vi "Browser.vi"() -> ()   [LabVIEW 2023, in "LV-Awesome.lvlib"]
uses:
  LV-Awesome.lvlib
  LV Awesome/LV Awesome.lvclass/LV Awesome.ctl
  Freetype Drawer/Freetype Drawer/Freetype Drawer.lvclass
  LV Awesome/Read Fonts.vi
  LV Awesome/Read Glyphs.vi
  Font Glyph Drawer Interface/Bitmap Canvas/Bitmap Canvas.lvclass
  LV Awesome/LV Awesome.lvclass
  Font Glyph Drawer Interface/Transform/Transform.lvclass
  Glyph .NET Drawer/Drawer .Net.lvclass
  Font Glyph Drawer Interface/Glyph Canvas/Glyph Canvas.lvclass
panel:
  out "To":i32
  out "From":i32
  in  "Exit":bool
  in  "Namespace":string(combo)
  in  "Combo Box":string(combo) caption="Search"
  out "Count":i32 caption="# Results"
  in  "Scrollbar":i32(c297)
  out "Icons":T1(array[cluster])
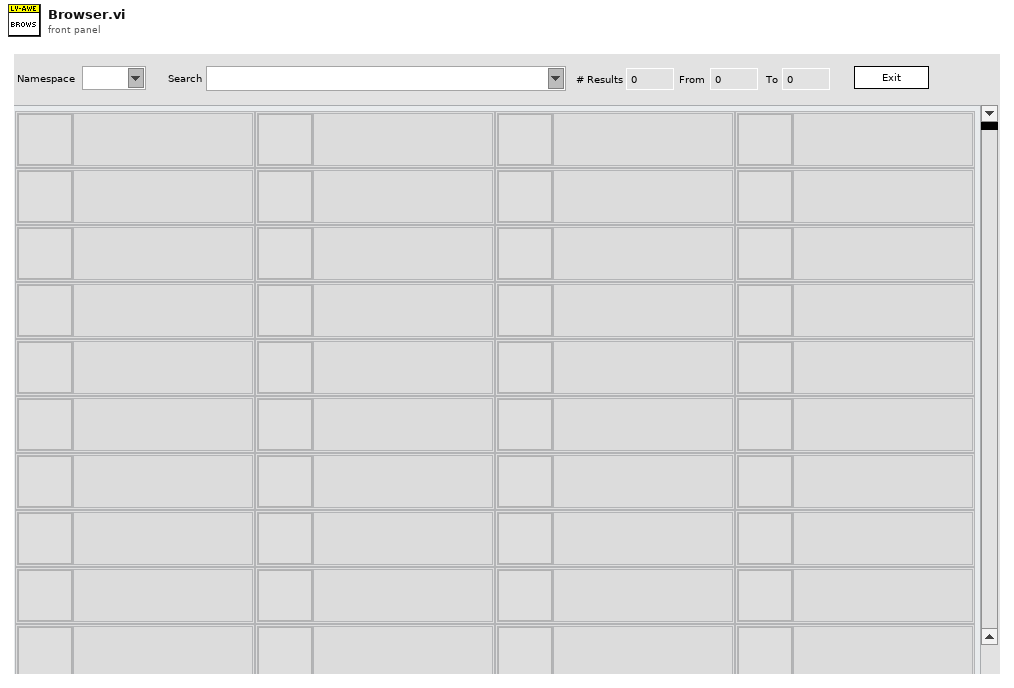
[diagram p1: front panel]
types:
  T1 = cluster{"2D Picture":picture, "String":string}[][]
  T2 = cluster{"Front":cluster{"Color":u32, "Alpha":u8}, "Back":cluster{"Color":u32, "Alpha":u8}}
  T3 = typedef "LVBoundsTypeDef.ctl" = cluster{"Width":u32, "Height":u32}
  T4 = cluster{"new picture":picture, "Glyph":string}[][]
  T5 = typedef "LVPoint32TypeDef.ctl" = cluster{"Horizontal":i32, "Vertical":i32}
  T6 = typedef "LVRowAndColumnTypeDef.ctl" = cluster{"Row":i32, "Column":i32}
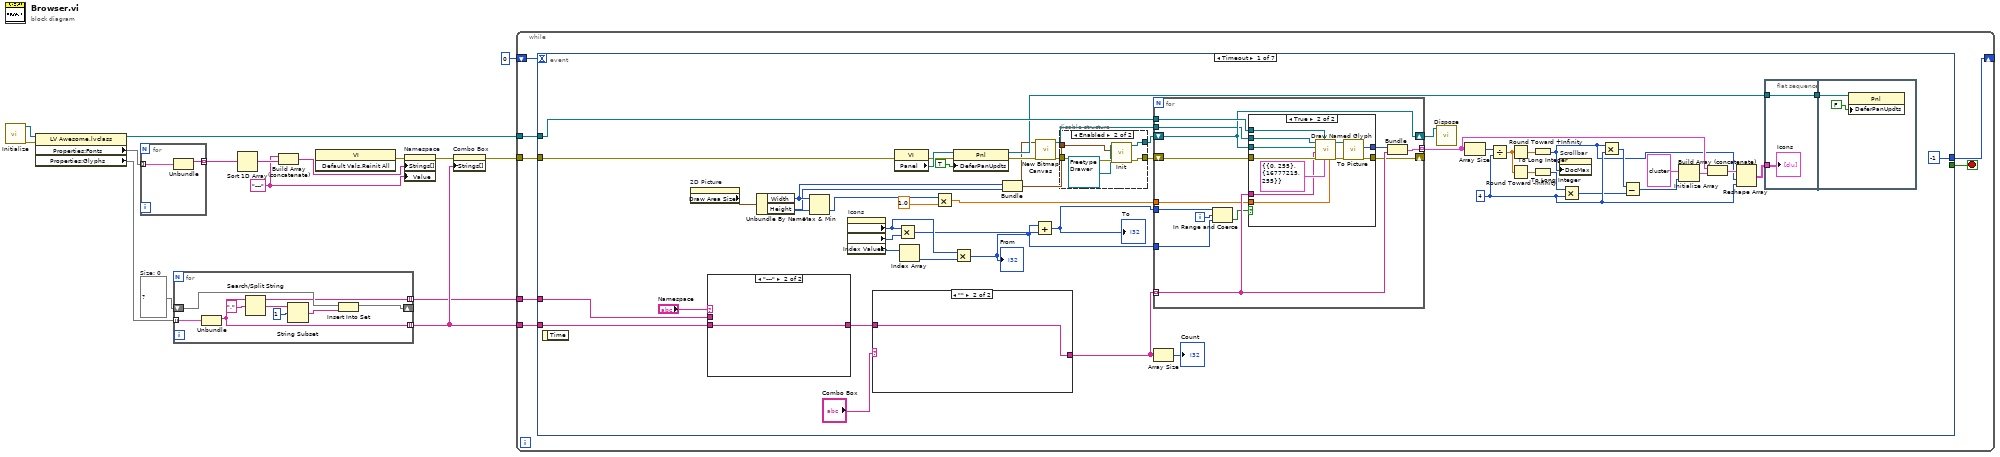
[diagram p0: block diagram]
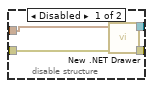
[diagram p2: hidden frame]
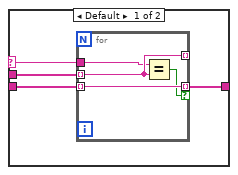
[diagram p3: hidden frame]
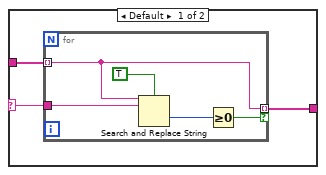
[diagram p4: hidden frame]
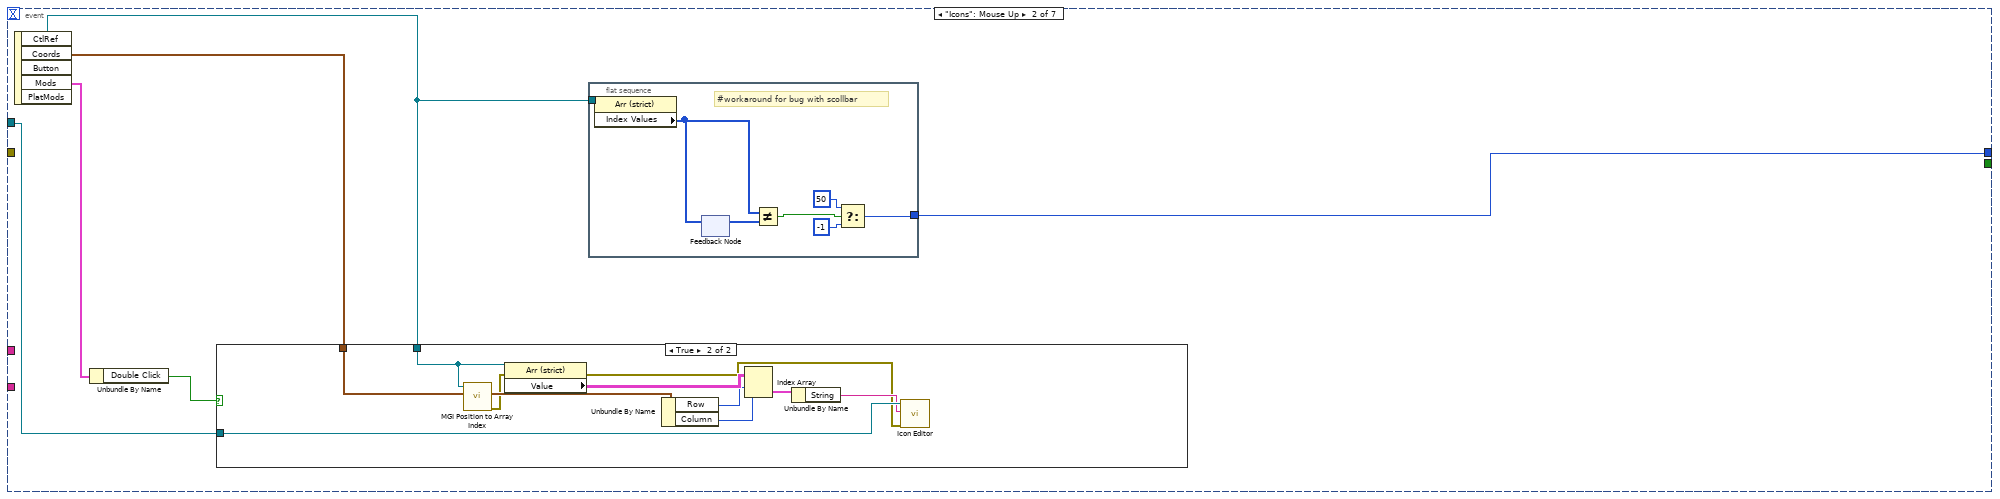
[diagram p6: hidden frame]
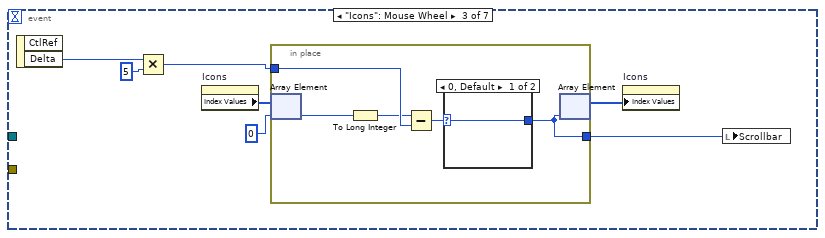
[diagram p8: hidden frame]
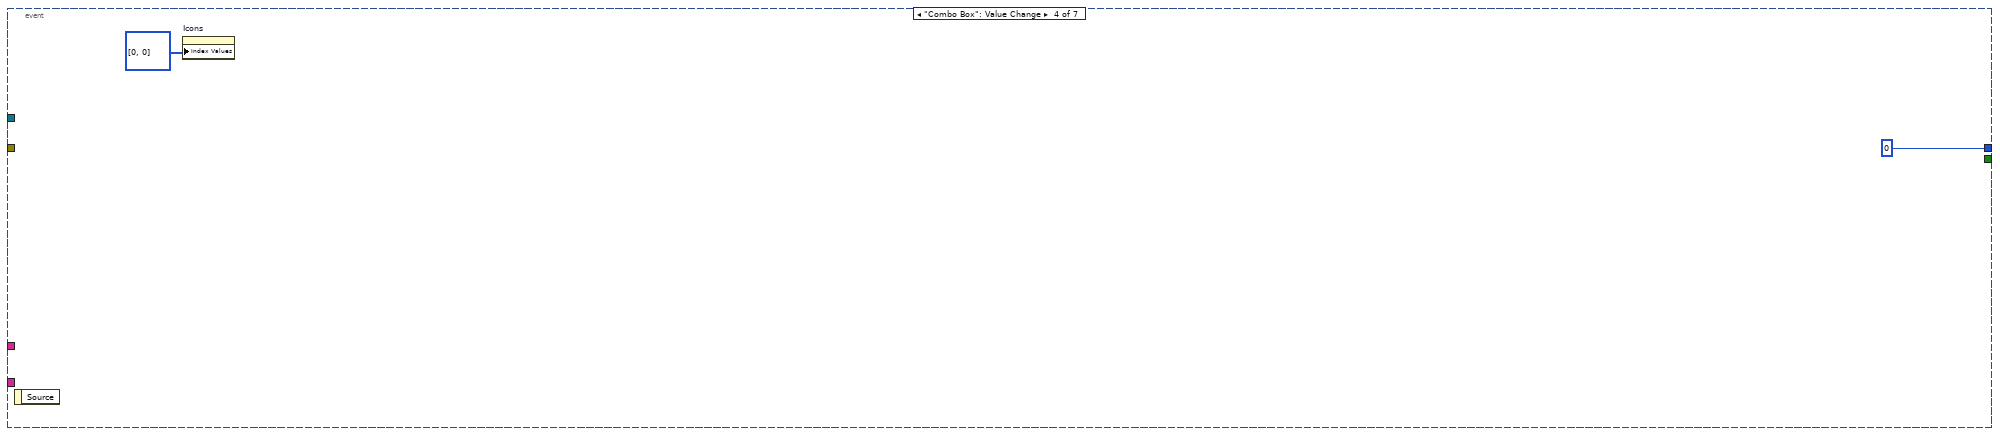
[diagram p10: hidden frame]
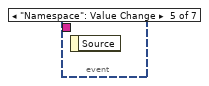
[diagram p11: hidden frame]
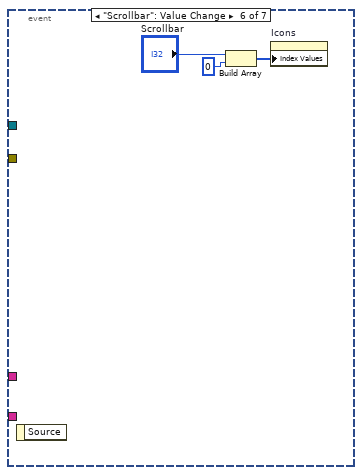
[diagram p12: hidden frame]
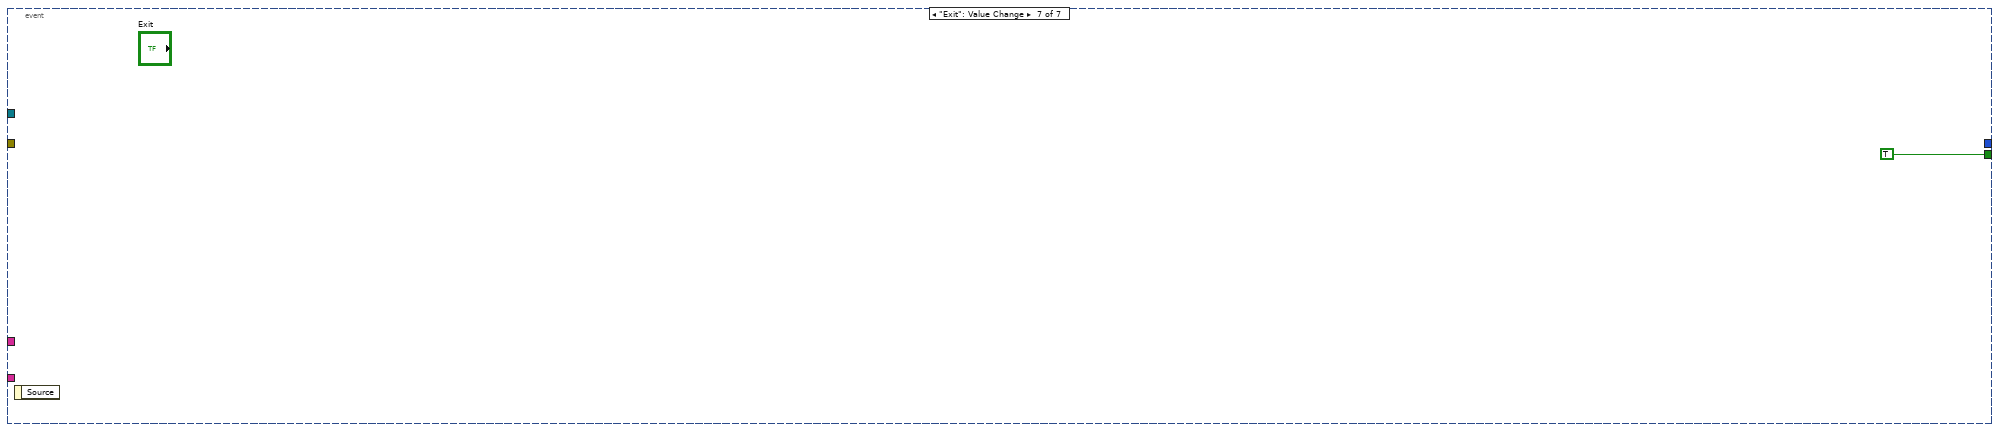
[diagram p13: hidden frame]
diagram:
  w8 = "---"
  w11 = set{string} {}  # Size: 0
  n1 = call "Initialize.vi"() -> ("error out"=w3:errorcluster, "LV Awesome"=w14:refnum<class "LV Awesome.lvclass">)  [unwired: 10 in]
  n2 = property class="LV Awesome.lvclass"(reference=w14, error in=w3) -> (reference out=w4:refnum<class "LV Awesome.lvclass">, "Properties:Fonts"=w2:map{string, path}, "Properties:Glyphs"=w1:map{string, u32})  [unwired: 1 out]
  n3 = for {
    tunnel: w2 -> [w18] mode=indexing
    tunnel: [w17] -> w13 mode=indexing
    n4 = Unbundle(w18) -> ("short"=w17:string)  [unwired: 1 out]
  }
  n5 = for {
    tunnel: w1 -> [w27] mode=indexing
    tunnel: [w26] -> w16 mode=indexing
    shift-right: [w21] -> _
    shift-left: w11 -> [w22]
    tunnel: [w19] -> w10 mode=indexing
    n6 = Unbundle(w27) -> ("Glyph"=w26:string)  [unwired: 1 out]
    n7 = Search/Split String(string=w26, search string/char (-)=".") -> (substring before match=w19:string, match + rest of string=w24:string)  [unwired: 1 in, 1 out]
    n8 = String Subset(string=w24, offset (0)=1) -> (substring=w20:string)  [unwired: 1 in]
    n9 = Insert Into Set(10:w20, 11:w22) -> (3:w21:set{string})  [unwired: 1 out]
  }
  n10 = Sort 1D Array(array=w13) -> (sorted array=w12:string[])
  n11 = Build Array (concatenate)(w8, w12) -> (w9:string[])
  n12 = invoke class="VI" method="Default Vals.Reinit All"() -> (error out=w7:errorcluster)  [unwired: 3 in, 2 out]
  n13 = property on="Namespace" class="CmbBox"(error in=w7, "Strings[]"=w9, "Value"=w8) -> (error out=w6:errorcluster)  [unwired: 1 in, 1 out]
  n14 = property on="Combo Box" class="CmbBox"(error in=w6, "Strings[]"=w16) -> (error out=w5:errorcluster)  [unwired: 1 in, 1 out]
  n15 = while {
    tunnel: w4 -> [w34]
    tunnel: w16 -> [w33]
    shift-right: [w31] -> _
    shift-left: 0 -> [w32]
    tunnel: w10 -> [w30]
    tunnel: w5 -> [w28]
    stop <- w29 stop-if-true
    n16 = event shown="[0] Timeout" {
      selector: _ -> [_ _ _ _ _ _ _]
      dyn-events: _ -> [_ _ _ _ _ _ _]
      timeout: w32 -> [_ _ _ _ _ _ _]
      tunnel: w34 -> [w84 w141 _ _ _ _ _]
      tunnel: w33 -> [w59 _ _ _ _ _ _]
      tunnel: [-1 w146 _ 0 _ _ _] -> w31
      tunnel: w30 -> [w57 _ _ _ _ _ _]
      tunnel: [_ _ _ _ _ _ TRUE] -> w29
      tunnel: w28 -> [w51 _ _ _ _ _ _]
      event Timeout {
        w66 = 4 ("y")
        n17 = event-data() -> ()  [unwired: 1 in, 1 out]
        n18 = property on="2D Picture" class="Pict"() -> ("Draw Area Size"=w40:T3)  [unwired: 2 in, 2 out]
        n19 = case shown="\"---\"" "Namespace" {
          selector: "Namespace" -> [w100 _]
          tunnel: w59 -> [w99 w106]
          tunnel: [w98 w106] -> w58
          tunnel: w57 -> [w101 _]
          frame Default {
            n20 = for {
              tunnel: [w105] -> _ mode=indexing
              tunnel: w101 -> [w105] mode=indexing
              tunnel: w100 -> [w104]
              tunnel: [w103] -> w98 mode=indexing if=w102
              tunnel: w99 -> [w103] mode=indexing
              n21 = Equal?(x=w104, y=w105) -> (x = y?=w102:bool)
            }
          }
          frame "---" {
          }
        }
        n22 = Unbundle By Name(w40) -> ("Width"=w36:u32, "Height"=w35:u32)
        n23 = Max & Min(x=w36, y=w35) -> (min(x,y)=w39:u32)  [unwired: 1 out]
        n24 = property on="Icons" class="Arr (strict)"() -> ("Number of Columns"=w78:u32, "Number of Rows"=w79:u32, "Index Values"=w81:u32[])  [unwired: 2 in, 2 out]
        n25 = case shown="\"\"" "Combo Box" {
          selector: "Combo Box" -> [w108 _]
          tunnel: w58 -> [w109 w115]
          tunnel: [w107 w115] -> w63
          frame Default {
            n26 = for {
              tunnel: w109 -> [w113] mode=indexing
              tunnel: w108 -> [w114]
              tunnel: [w113] -> w107 mode=indexing if=w111
              n27 = Search and Replace String(case sensitive?=TRUE ("ignore case? (F)"), input string=w113, search string=w114) -> (offset past replacement=w112:i32)  [unwired: 5 in, 3 out]
              n28 = Greater Or Equal To 0?(x=w112) -> (x >= 0?=w111:bool)
            }
          }
          frame "" {
          }
        }
        n29 = property class="VI"(error in=w51) -> (error out=w48:errorcluster, "Panel"=w50:refnum<vi>)  [unwired: 1 in, 1 out]
        n30 = Multiply(x=w78, y=w79) -> (x*y=w77:u32)
        n31 = Index Array(array=w81) -> (element=w80:u32)  [unwired: 1 in]
        n32 = Multiply(x=w39, y=1.0) -> (x*y=w38:dbl)
        n33 = property class="Pnl"(reference=w50, error in=w48, "DeferPanUpdts"=TRUE ("Defer Panel Updates")) -> (reference out=w44:refnum<vi>, error out=w47:errorcluster)
        n34 = Multiply(x=w78, y=w80) -> (x*y=w54:u32)
        "From" <- w54
        n35 = Bundle("Width"=w36, "Height"=w35) -> (w41:cluster{"Width":u32, "Height":u32})  [unwired: 1 in]
        n36 = Add(x=w54, y=w77) -> (x+y=w53:u32)
        "To" <- w53
        n37 = call "New Bitmap Canvas.vi"("error in (no error)"=w47, "Size"=w41) -> ("error out"=w46:errorcluster, "Bitmap Canvas out"=w52:refnum<class "Bitmap Canvas.lvclass">)  [unwired: 8 in]
        n38 = disable-structure shown="Enabled" {
          disable-tunnel: [w88 w90] -> w62
          disable-tunnel: w46 -> [w87 w93]
          disable-tunnel: [w86 w92] -> w45
          disable-tunnel: w41 -> [w85 w89]
          frame Disabled {
            n39 = call "New .NET Drawer.vi"("error in (no error)"=w87, "Size"=w85) -> ("error out"=w86:errorcluster, "Canvas out"=w88:refnum<class "Drawer .Net.lvclass">)  [unwired: 8 in]
          }
          frame Enabled {
            n40 = call-dynamic "Init.vi"("error in (no error)"=w93, "Size"=w89, "Class 1 in"=refnum<class "Freetype Drawer.lvclass"> refnum ("Freetype Drawer.lvlib:Freetype Drawer.lvclass")) -> ("error out"=w92:errorcluster, "Class 1 out"=w90:refnum<class "Freetype Drawer.lvclass">)  [unwired: 7 in]
          }
        }
        n41 = for {
          tunnel: [w127] -> w76 mode=indexing
          tunnel: w84 -> [w126]
          tunnel: w63 -> [w125] mode=indexing
          tunnel: w54 -> [w122]
          tunnel: w53 -> [w121]
          tunnel: w38 -> [w119]
          tunnel: w52 -> [w118]
          shift-right: [w117] -> _
          shift-left: w45 -> [w116]
          shift-right: [w124] -> w61
          shift-left: w62 -> [w124]
          i -> [w123]
          n42 = In Range and Coerce(upper limit=w121, x=w123, lower limit=w122) -> (In Range?=w120:bool)  [unwired: 1 out]
          n43 = case shown="True" w120 {
            tunnel: [_ w140] -> w128
            tunnel: w126 -> [_ w133]
            tunnel: w125 -> [_ w132]
            tunnel: w124 -> [_ w139]
            tunnel: w119 -> [_ w130]
            tunnel: w118 -> [_ w138]
            tunnel: [w129 w137] -> w117
            tunnel: w116 -> [w129 w134]
            frame False {
            }
            frame True {
              n44 = call "Draw Named Glyph.vi"("Size"=w130, "Colors"=T2 {"Front"={"Color"=0, "Alpha"=255}, "Back"={"Color"=16777215, "Alpha"=255}}, "Glyph Source in"=w133, "error in (no error)"=w134, "Glyph Name"=w132, "Glyph Drawer in"=w139, "Glyph Canvas in"=w138) -> ("error out"=w136:errorcluster, "Glyph Canvas out"=w131:refnum<class "Bitmap Canvas.lvclass">)  [unwired: 2 in, 1 out]
              n45 = call "To Picture.vi"("error in (no error)"=w136, "Bitmap Canvas in"=w131) -> ("error out"=w137:errorcluster, "new picture"=w140:picture)  [unwired: 7 in, 1 out]
            }
          }
          n46 = Bundle("new picture"=w128, "Glyph"=w125) -> (w127:cluster{"new picture":picture, "Glyph":string})  [unwired: 1 in]
        }
        n47 = Array Size(array=w63) -> (size(s)=→"Count":i32)
        n48 = call-dynamic "Dispose.vi"("Class 1 in"=w61) -> ()  [unwired: 10 in, 1 out]
        n49 = Array Size(array=w76) -> (size(s)=w75:i32)
        n50 = Divide(x=w75, y=w66) -> (x/y=w69:dbl)
        n51 = Round Toward +Infinity(x=w69) -> (ceil(x): smallest int >= x=w70:dbl)
        n52 = Round Toward -Infinity(1:w69) -> (0:w68:dbl)
        n53 = To Long Integer(number=w70) -> (32bit integer=w55:i32)
        n54 = To Long Integer(number=w68) -> (32bit integer=w67:i32)
        n55 = property on="Scrollbar" class="Scroll (strict)"("DocMax"=w55) -> ()  [unwired: 2 in, 2 out]
        n56 = Multiply(x=w67, y=w66) -> (x*y=w64:i32)
        n57 = Multiply(x=w55, y=w66) -> (x*y=w65:i32)
        n58 = Subtract(x=w65, y=w64) -> (x-y=w71:i32)
        n59 = Initialize Array(cluster{"new picture":picture, "Glyph":string} {"new picture"=bytes[0], "Glyph"=""}, w71) -> (w72:cluster{"new picture":picture, "Glyph":string}[])
        n60 = Build Array (concatenate)(w76, w72) -> (w73:cluster{"new picture":picture, "Glyph":string}[])
        n61 = Reshape Array(w73, w55, w66) -> (w42:T4)
        n62 = flat-sequence {
          tunnel: w44 -> [w95]
          tunnel: [w95] -> w43
          tunnel: w42 -> [w94]
          tunnel: w43 -> [w97]
          frame #0 {
            "Icons" <- w94
          }
          frame #1 {
            n63 = property class="Pnl"(reference=w97, "DeferPanUpdts"=FALSE ("Defer Panel Updates")) -> ()  [unwired: 1 in, 2 out]
          }
        }
      }
      event "Icons": Mouse Up {
        n64 = event-data() -> ("CtlRef"=w144:refnum<vi>, "Coords"=w142:T5, "Mods"=w145:cluster{"Double Click":bool, "Menu Key":bool})  [unwired: 1 in, 2 out]
        n65 = Unbundle By Name(w145) -> ("Double Click"=w143:bool)
        n66 = case shown="True" w143 {
          tunnel: w144 -> [_ w155]
          tunnel: w142 -> [_ w157]
          tunnel: w141 -> [_ w150]
          frame False {
          }
          frame True {
            n67 = call <userlib>:"MGI Position to Array Index.vi"("Coords"=w157, "ArrayRef"=w155) -> ("error out"=w147:errorcluster, "Index"=w156:T6)  [unwired: 5 in, 3 out]
            n68 = property class="Arr (strict)"(reference=w155, error in=w147) -> (error out=w148:errorcluster, "Value"=w154:T1)  [unwired: 1 out]
            n69 = Unbundle By Name(w156) -> ("Row"=w153:i32, "Column"=w152:i32)
            n70 = Index Array(array=w154, index (row)=w153, index (col)=w152) -> (element=w151:cluster{"2D Picture":picture, "String":string})
            n71 = Unbundle By Name(w151) -> ("String"=w149:string)
            n72 = call "Icon Editor.vi"("error in (no error)"=w148, "Glyph"=w149, "Glyph Source in"=w150) -> ()  [unwired: 7 in, 2 out]
          }
        }
        n73 = flat-sequence {
          tunnel: w144 -> [w164]
          tunnel: [w163] -> w146
          frame #0 {
            # "#workaround for bug with scollbar"
            n74 = property class="Arr (strict)"(reference=w164) -> ("Index Values"=w161:u32[])  [unwired: 1 in, 2 out]
            n75 = feedback #1() -> (w162:u32[])  [unwired: 1 in]
            n76 = feedback-in #1(w161) -> ()
            n77 = Not Equal?(x=w161, y=w162) -> (x != y?=w159:bool)
            n78 = Select(t=50, s=w159, f=-1) -> (s? t:f=w163:i32)
          }
        }
      }
      event "Icons": Mouse Wheel {
        n79 = event-data() -> ("Delta"=w171:i32)  [unwired: 1 in, 1 out]
        n80 = Multiply(x=w171, y=5) -> (x*y=w167:i32)
        n81 = property on="Icons" class="Arr (strict)"() -> ("Index Values"=w170:u32[])  [unwired: 2 in, 2 out]
        n82 = in-place {
          in-place-border: w167 -> [w175]
          in-place-border: [w172] -> w165
          n83 = in-place-array #2(w170, 0) -> (w176:u32)
          n84 = To Long Integer(number=w176) -> (32bit integer=w174:i32)
          n85 = Subtract(x=w174, y=w175) -> (x-y=w173:i32)
          n86 = case shown="0, Default" w173 {
            selector: w173 -> [w177 _]
            tunnel: [w177 _] -> w172
            frame 0, Default {
            }
            frame ..-1 {
            }
          }
          n87 = in-place-array #2(w172) -> (w169:u32[])  [unwired: 1 out]
        }
        n88 = property on="Icons" class="Arr (strict)"("Index Values"=w169) -> ()  [unwired: 2 in, 2 out]
        n89 = local write "Scrollbar"(w165) -> ()
      }
      event "Combo Box": Value Change {
        n90 = event-data() -> ()  [unwired: 1 in, 1 out]
        n91 = property on="Icons" class="Arr (strict)"("Index Values"=u32[] [0, 0]) -> ()  [unwired: 2 in, 2 out]
      }
      event "Namespace": Value Change {
        n92 = event-data() -> ()  [unwired: 1 in, 1 out]
      }
      event "Scrollbar": Value Change {
        n93 = event-data() -> ()  [unwired: 1 in, 1 out]
        n94 = Build Array("Scrollbar", 0 ("element")) -> (w180:i32[])
        n95 = property on="Icons" class="Arr (strict)"("Index Values"=w180) -> ()  [unwired: 2 in, 2 out]
      }
      event "Exit": Value Change {
        n96 = event-data() -> ()  [unwired: 1 in, 1 out]
      }
    }
  }
